vi "_consumeToken.vi"(8 "error in (no error)":errorcluster, 11 "JSON Parser In":refnum<class "tJSONParser.lvclass">) -> (0 "error out":errorcluster, 3 "JSON Parser Out":refnum<class "tJSONParser.lvclass">)   [LabVIEW 2013, in "JSON.lvlib" / "tJSONParser.lvclass"]
doc: "Consumes the next token and sets the token type on the JSONParser object."
uses:
  tJSONParser.lvclass
  tJSONParser.lvclass/tJSONParser.ctl
  _tokenType.ctl
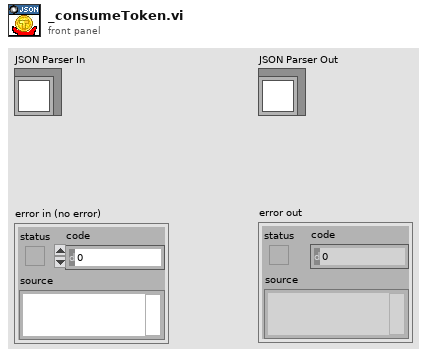
[diagram p1: front panel]
types:
  T1 = typedef "JSON.lvlib/tJSONParser.lvclass/_tokenType.ctl" = enum16{"Object Begin", "Object End", "Array Begin", "Array End", "String Delimeter", "Forward Slash", "Number", "Boolean", "Null", "Object Or Array Separator", "Pair Separator", "End Of File", "Asterisk", "Backward Slash", "Other"}
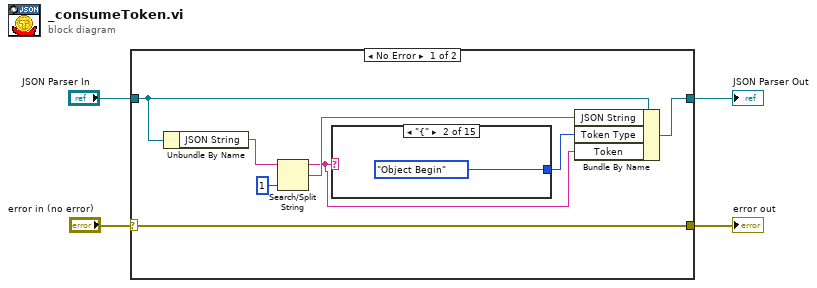
[diagram p0: block diagram]
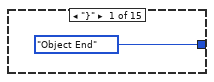
[diagram p2: hidden frame]
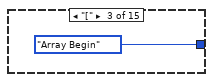
[diagram p3: hidden frame]
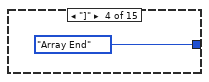
[diagram p4: hidden frame]
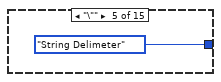
[diagram p5: hidden frame]
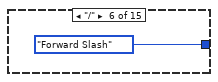
[diagram p6: hidden frame]
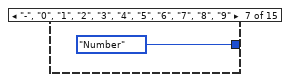
[diagram p7: hidden frame]
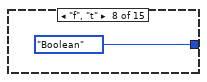
[diagram p8: hidden frame]
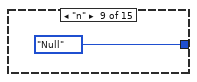
[diagram p9: hidden frame]
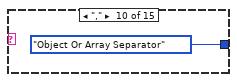
[diagram p10: hidden frame]
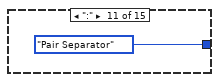
[diagram p11: hidden frame]
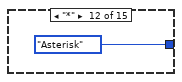
[diagram p12: hidden frame]
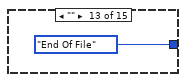
[diagram p13: hidden frame]
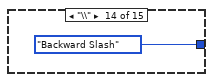
[diagram p14: hidden frame]
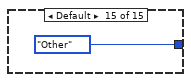
[diagram p15: hidden frame]
diagram:
  n1 = case shown="No Error" "error in (no error)" {
    selector: "error in (no error)" -> [w12 w29]
    tunnel: [w12 w29] -> w3
    tunnel: "JSON Parser In" -> [w11 w28]
    tunnel: [w6 w28] -> w1
    frame No Error {
      n2 = Unbundle By Name(w11) -> ("JSON String"=w7:string)
      n3 = Search/Split String(string=w7, offset (0)=1) -> (substring before match=w5:string, match + rest of string=w8:string)  [unwired: 1 in, 1 out]
      n4 = case shown="\"{\"" w5 {
        tunnel: [_tokenType."Object End" ("Token Type") _tokenType."Object Begin" ("Token Type") _tokenType."Array Begin" ("Token Type") _tokenType."Array End" ("Token Type") _tokenType."String Delimeter" ("Token Type") _tokenType."Forward Slash" ("Token Type") _tokenType."Number" ("Token Type") _tokenType."Boolean" ("Token Type") _tokenType."Null" ("Token Type") _tokenType."Object Or Array Separator" ("Token Type") _tokenType."Pair Separator" ("Token Type") _tokenType."Asterisk" ("Token Type") _tokenType."End Of File" ("Token Type") _tokenType."Backward Slash" ("Token Type") _tokenType."Other" ("Token Type")] -> w10
        frame "}" {
        }
        frame "{" {
        }
        frame "[" {
        }
        frame "]" {
        }
        frame "\"" {
        }
        frame "/" {
        }
        frame "-", "0", "1", "2", "3", "4", "5", "6", "7", "8", "9" {
        }
        frame "f", "t" {
        }
        frame "n" {
        }
        frame "," {
        }
        frame ":" {
        }
        frame "*" {
        }
        frame "" {
        }
        frame "\\" {
        }
        frame Default {
        }
      }
      n5 = Bundle By Name(cluster=w11, "JSON String"=w8, "Token Type"=w10, "Token"=w5) -> (w6:refnum<class "tJSONParser.lvclass">)
    }
    frame Error {
    }
  }
  "error out" <- w3
  "JSON Parser Out" <- w1
